vi "Write FileHeader.vi"(10 "FileHeader":refnum<class "FileHeader.lvclass">, 11 "ConfigManager.Text in":refnum<class "ConfigManager.Text.lvclass">) -> (3 "ConfigManager.Text out":refnum<class "ConfigManager.Text.lvclass">)   [LabVIEW 2013, in "CfgManager.Text.lvlib" / "ConfigManager.Text.lvclass"]
uses:
  ConfigManager.Text.lvclass
  FileHeader/FileHeader.lvclass
  ConfigManager.Text.lvclass/ConfigManager.Text.ctl
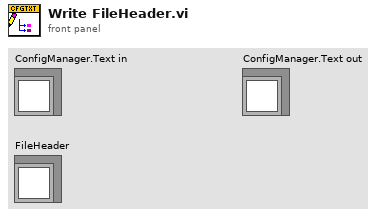
[diagram p1: front panel]
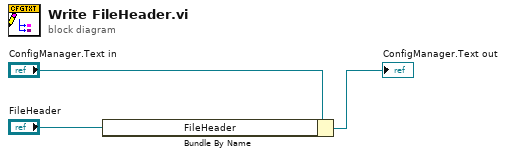
[diagram p0: block diagram]
diagram:
  n1 = Bundle By Name(cluster="ConfigManager.Text in", "FileHeader"="FileHeader") -> (→"ConfigManager.Text out":refnum<class "ConfigManager.Text.lvclass">)
